vi "XML Read Variables.vi"(10 "XML Result":string, 11 "XML Worksheet":string="<worksheet xmlns:xsi=\"http://www.w3.org/2001/XMLSchema-instance\" xmlns:ve=\"http://schemas.openxmlformats.org/markup-compatibility/2006\" xmlns:r=\"http://schemas.openxmlformats.org/officeDocument/2006/relationships\" xmlns:ws=\"http://schemas.mathsoft.com/worksheet50\" xmlns:ml=\"http://schemas.mathsoft.com/math50\" xmlns:u=\"http://schemas.mathsoft.com/units10\" xmlns:p=\"http://schemas.mathsoft.com/provenance10\" xmlns=\"http://schemas.mathsoft.com/worksheet50\"><regions><region region-id=\"0\" top=\"115.20000000000002\" left=\"0\"><math resultRef=\"0\"><ml:define><ml:id labels=\"VARIABLE\" xml:space=\"preserve\">QPlant</ml:id><ml:apply><ml:scale /><ml:real>4</ml:real><ml:apply><ml:div /><ml:id labels=\"UNIT\" label-is-contextual=\"true\" xml:space=\"preserve\">L</ml:id><ml:id labels=\"UNIT\" label-is-contextual=\"true\" xml:space=\"preserve\">s</ml:id></ml:apply></ml:apply></ml:define><resultFormat><matrix size=\"12,12\" offset=\"0,0\" show-indices=\"false\" expand-nested-arrays=\"false\" /></resultFormat></math></region><region region-id=\"1\" top=\"134.40000000000003\" left=\"249.60000000000002\"><math resultRef=\"2\"><ml:define><ml:id labels=\"VARIABLE\" xml:space=\"preserve\">Distance</ml:id><ml:apply><ml:scale /><ml:real>5.65</ml:real><ml:id labels=\"UNIT\" label-is-contextual=\"true\" xml:space=\"preserve\">m</ml:id></ml:apply></ml:define></math></region><region region-id=\"2\" top=\"172.8\" left=\"0\"><math resultRef=\"4\"><ml:define><ml:id labels=\"VARIABLE\" xml:space=\"preserve\">Flow</ml:id><ml:apply><ml:scale /><ml:real>6</ml:real><ml:apply><ml:div /><ml:id labels=\"UNIT\" label-is-contextual=\"true\" xml:space=\"preserve\">L</ml:id><ml:id labels=\"UNIT\" label-is-contextual=\"true\" xml:space=\"preserve\">s</ml:id></ml:apply></ml:apply></ml:define></math></region><region region-id=\"3\" top=\"211.20000000000005\" left=\"0\"><math resultRef=\"6\"><ml:define><ml:id labels=\"VARIABLE\" xml:space=\"preserve\">Area</ml:id><ml:apply><ml:scale /><ml:real>1</ml:real><ml:apply><ml:pow /><ml:id labels=\"UNIT\" label-is-contextual=\"true\" xml:space=\"preserve\">m</ml:id><ml:real>2</ml:real></ml:apply></ml:apply></ml:define></math></region><region region-id=\"4\" top=\"249.60000000000002\" left=\"0\"><math resultRef=\"8\"><ml:define><ml:id labels=\"VARIABLE\" xml:space=\"preserve\">Velocity</ml:id><ml:eval><ml:apply><ml:div /><ml:id labels=\"VARIABLE\" label-is-contextual=\"true\" xml:space=\"preserve\">Flow</ml:id><ml:id labels=\"VARIABLE\" label-is-contextual=\"true\" xml:space=\"preserve\">Area</ml:id></ml:apply><ml:unitOverride><ml:apply><ml:div /><ml:id labels=\"UNIT\" xml:space=\"preserve\">mm</ml:id><ml:id labels=\"UNIT\" xml:space=\"preserve\">s</ml:id></ml:apply></ml:unitOverride></ml:eval></ml:define></math></region><region region-id=\"5\" top=\"307.20000000000005\" left=\"0\"><math resultRef=\"10\"><ml:eval><ml:id labels=\"VARIABLE\" label-is-contextual=\"true\" xml:space=\"preserve\">Velocity</ml:id><ml:unitOverride><ml:placeholder /></ml:unitOverride></ml:eval></math></region><region region-id=\"6\" top=\"307.20000000000005\" left=\"230.40000000000003\"><math resultRef=\"12\"><ml:eval><ml:id labels=\"VARIABLE\" label-is-contextual=\"true\" xml:space=\"preserve\">QPlant</ml:id><ml:unitOverride><ml:placeholder /></ml:unitOverride></ml:eval></math></region><region region-id=\"7\" top=\"364.80000000000007\" left=\"0\"><math resultRef=\"14\"><ml:define><ml:id labels=\"VARIABLE\" xml:space=\"preserve\">QPlantOut</ml:id><ml:apply><ml:scale /><ml:real>2</ml:real><ml:id labels=\"VARIABLE\" label-is-contextual=\"true\" xml:space=\"preserve\">QPlant</ml:id></ml:apply></ml:define></math></region><region region-id=\"8\" top=\"364.80000000000007\" left=\"249.60000000000002\"><math resultRef=\"16\"><ml:define><ml:id labels=\"VARIABLE\" xml:space=\"preserve\">QPlantOutAgain</ml:id><ml:apply><ml:scale /><ml:real>3</ml:real><ml:id labels=\"VARIABLE\" label-is-contextual=\"true\" xml:space=\"preserve\">QPlant</ml:id></ml:apply></ml:define></math></region><region region-id=\"9\" top=\"422.40000000000009\" left=\"0\"><math resultRef=\"18\"><ml:define><ml:id labels=\"VARIABLE\" xml:space=\"preserve\">QOut</ml:id><ml:apply><ml:scale /><ml:real>3</ml:real><ml:id labels=\"VARIABLE\" label-is-contextual=\"true\" xml:space=\"preserve\">QPlant</ml:id></ml:apply></ml:define></math></region><region region-id=\"10\" top=\"499.20000000000005\" left=\"0\"><math resultRef=\"20\"><ml:eval><ml:id labels=\"VARIABLE\" label-is-contextual=\"true\" xml:space=\"preserve\">QOut</ml:id><ml:unitOverride><ml:placeholder /></ml:unitOverride></ml:eval></math></region><region region-id=\"11\" top=\"576.00000000000011\" left=\"19.200000000000003\"><math resultRef=\"22\"><ml:eval><ml:id labels=\"VARIABLE\" label-is-contextual=\"true\" xml:space=\"preserve\">QPlantOut</ml:id><ml:unitOverride><ml:placeholder /></ml:unitOverride></ml:eval></math></region><region region-id=\"12\" top=\"633.60000000000014\" left=\"19.200000000000003\"><math resultRef=\"24\"><ml:eval><ml:id labels=\"VARIABLE\" xml:space=\"preserve\">QPlantOutAgain</ml:id><ml:unitOverride><ml:apply><ml:div /><ml:id labels=\"UNIT\" xml:space=\"preserve\">L</ml:id><ml:id labels=\"UNIT\" xml:space=\"preserve\">s</ml:id></ml:apply></ml:unitOverride></ml:eval></math></region><region region-id=\"13\" top=\"729.60000000000014\" left=\"19.200000000000003\"><math resultRef=\"26\"><ml:define><ml:id labels=\"VARIABLE\" xml:space=\"preserve\">DoubleDistance</ml:id><ml:apply><ml:scale /><ml:real>2</ml:real><ml:id labels=\"VARIABLE\" label-is-contextual=\"true\" xml:space=\"preserve\">Distance</ml:id></ml:apply></ml:define></math></region><region region-id=\"14\" top=\"768.00000000000011\" left=\"19.200000000000003\"><math resultRef=\"28\"><ml:eval><ml:id labels=\"VARIABLE\" xml:space=\"preserve\">DoubleDistance</ml:id><ml:unitOverride><ml:placeholder /></ml:unitOverride></ml:eval></math></region></regions></worksheet>") -> (3 "Variable Clusters out":T1)   [LabVIEW 2011, in "Design Server.lvlib"]
uses:
  Design Server.lvlib
  Variable cluster.ctl
panel:
  out "Contents":string[](array[string])
  out "Results":string[](array[string])
  out "Result ID":i32[](array[numeric])
  out "Name.Sub":string[](array[string])
  out "Worksheet ID":i32[](array[numeric])
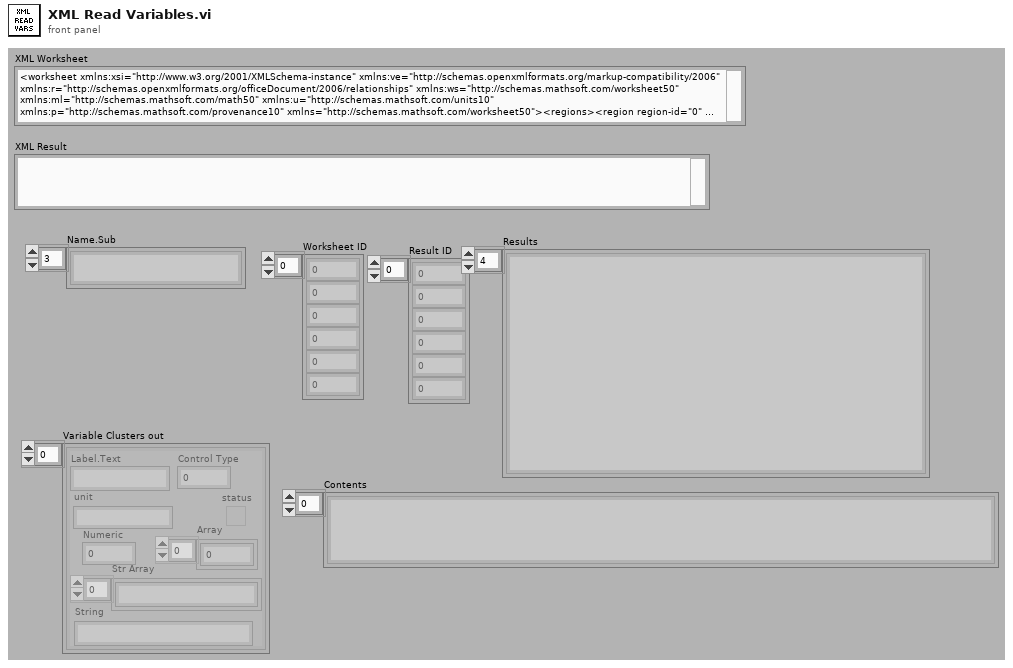
[diagram p1: front panel]
types:
  T1 = typedef "Design Server.lvlib/Variable cluster.ctl" = cluster{"Label.Text":string, "Control Type":u32, "Numeric":dbl, "Array":dbl[], "status":bool, "Str Array":string[], "String":string, "unit":string}[]
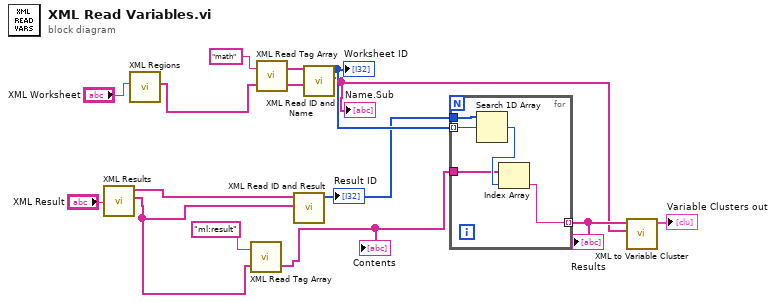
[diagram p0: block diagram]
diagram:
  n1 = call "XML Results.vi"("XML"="XML Result") -> ("XML content"=w7:string[], "Tag parameters"=w8:string[])  [unwired: 8 in]
  n2 = call "XML Regions.vi"("XML"="XML Worksheet") -> ("XML content"=w13:string[])  [unwired: 8 in, 1 out]
  n3 = call "XML Read Tag Array.vi"("XML content"=w7, "XML Tag"="ml:result") -> ("Contents"=w4:string[])  [unwired: 1 out]
  "Contents" <- w4
  n4 = call "XML Read Tag Array.vi"("XML content"=w13, "XML Tag"="math") -> ("Contents"=w9:string[], "Tags"=w10:string[])
  n5 = call "XML Read ID and Result.vi"("Result Contents"=w7, "Result Tags"=w8) -> ("Result ID"=w5:i32[])  [unwired: 8 in, 1 out]
  "Result ID" <- w5
  n6 = call "XML Read ID and Name.vi"("Math Contents"=w9, "Math Tags"=w10) -> ("Name.Sub"=w2:string[], "Result ID"=w6:i32[])  [unwired: 8 in]
  "Worksheet ID" <- w6
  "Name.Sub" <- w2
  n7 = for {
    tunnel: w6 -> [w20] mode=indexing
    tunnel: w5 -> [w19]
    tunnel: w4 -> [w17]
    tunnel: [w16] -> w3 mode=indexing
    n8 = Search 1D Array(1D array=w19, element=w20) -> (index of element=w18:i32)  [unwired: 1 in]
    n9 = Index Array(array=w17, index=w18) -> (element=w16:string)
  }
  "Results" <- w3
  n10 = call "XML to Variable Cluster.vi"("Name.Sub"=w2, "After Var Name"=w3) -> ("Variable Clusters out"=→"Variable Clusters out":T1)  [unwired: 9 in]
